vi "Generate ServiceImpl Class.vi"(7 "RPC Method Parameters":T1[](array[typedef]), 8 "error in (no error)":errorcluster, 10 "Service base class in":refnum<vi>, 11 "UserCode Lib in":refnum<vi>) -> (0 "error out":errorcluster, 2 "Service Impl class out":refnum<vi>, 3 "Service Base class out":refnum<vi>)   [LabVIEW 2019, in "gRPC Template Creation Utility.lvlib"]
uses:
  gRPC Template Creation Utility.lvlib
  TypeDefs/RPC Method Parameters.ctl
panel:
  out "UserCode Lib out":refnum<vi>
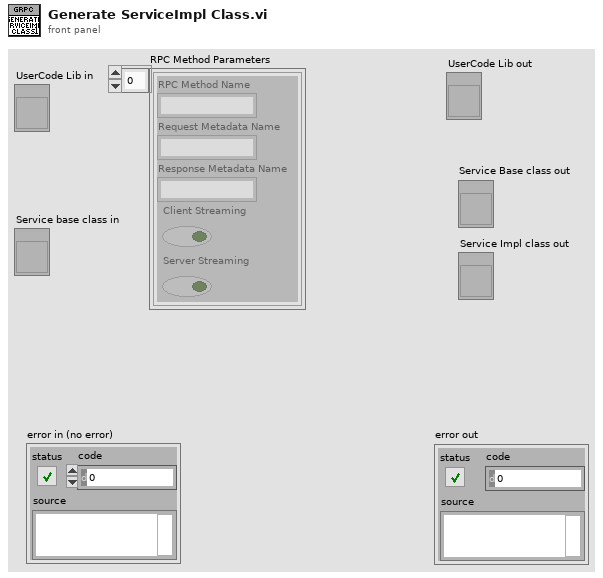
[diagram p1: front panel]
types:
  T1 = typedef "gRPC Template Creation Utility.lvlib/RPC Method Parameters.ctl" = cluster{"RPC Method Name":string, "Request Metadata Name":string, "Response Metadata Name":string, "Client Streaming":bool, "Server Streaming":bool}
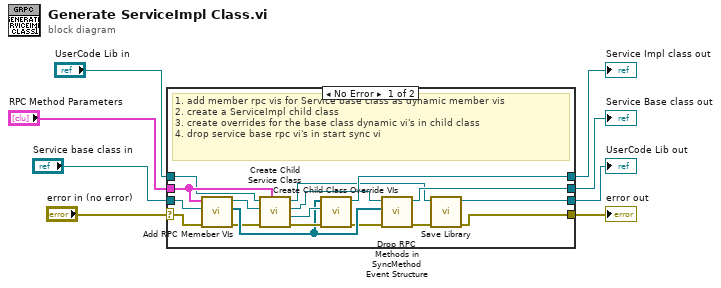
[diagram p0: block diagram]
diagram:
  n1 = case shown="No Error" "error in (no error)" {
    selector: "error in (no error)" -> [w24 w28]
    tunnel: [w13 w28] -> w7
    tunnel: "Service base class in" -> [w25 w27]
    tunnel: [w15 w27] -> w5
    tunnel: "RPC Method Parameters" -> [w23 _]
    tunnel: "UserCode Lib in" -> [w10 w26]
    tunnel: [w9 w26] -> w2
    tunnel: [w20 _] -> w1
    frame No Error {
      # "1. add member rpc vis for Service base class as dynamic member vis\n2. create a ServiceImpl child class\n3. create overrides for the base class dynamic vi's in child class\n4. drop service base rpc vi's in start sync vi"
      n2 = call "Add RPC Memeber VIs.vi"("error in"=w24, "LVClassLibrary in"=w25, "RPC Method Parameters"=w23) -> ("error out"=w11:errorcluster, "Dynamic member VIs"=w17:refnum<vi>[], "LVClassLibrary out"=w22:refnum<vi>)  [unwired: 6 in]
      n3 = call "Create Child Service Class.vi"("RPC Method Parameters"=w23, "error in (no error)"=w11, "Service base class in"=w22, "Server Library in"=w10) -> ("error IO"=w19:errorcluster, "Service Impl class out"=w21:refnum<vi>, "Service base class out"=w18:refnum<vi>, "Server Library out"=w12:refnum<vi>)  [unwired: 4 in]
      n4 = call "Create Child Class Override VIs.vi"("error in"=w19, "Service Impl class in"=w21, "base class dynamic member VIs"=w17) -> ("error out"=w16:errorcluster, "Service Impl class out"=w20:refnum<vi>)  [unwired: 7 in]
      n5 = call "Drop RPC Methods in SyncMethod Event Structure.vi"("error in (no error)"=w16, "dynamic member VIs"=w17, "Server class in"=w18) -> ("error out"=w14:errorcluster, "Server class out"=w15:refnum<vi>)  [unwired: 7 in]
      n6 = call "Save Library.vi"("error in (no error)"=w14, "Library in"=w12) -> ("error out"=w13:errorcluster, "Library out"=w9:refnum<vi>)  [unwired: 8 in]
    }
    frame Error {
    }
  }
  "error out" <- w7
  "Service Base class out" <- w5
  "UserCode Lib out" <- w2
  "Service Impl class out" <- w1
